vi "ErrorDialog.vi"(8 "error in":errorcluster) -> (0 "error out":errorcluster)   [LabVIEW 2010]
panel:
  out "Message":string
  in  "OK":bool
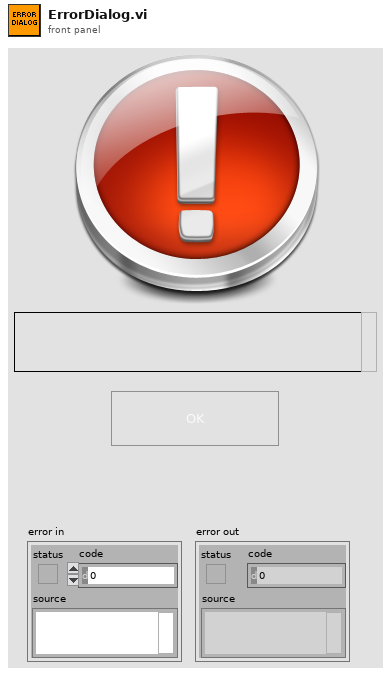
[diagram p1: front panel]
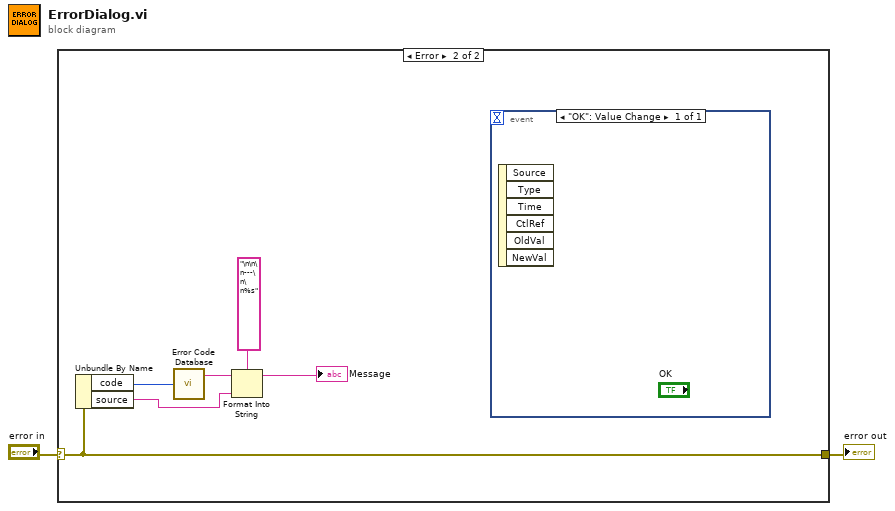
[diagram p0: block diagram]
diagram:
  n1 = case shown="Error" "error in" {
    selector: "error in" -> [w3 w9]
    tunnel: [w3 w9] -> w1
    frame No Error {
    }
    frame Error {
      n2 = Unbundle By Name(w9) -> ("code"=w8:i32, "source"=w4:string)
      n3 = call <vilib>:"Error Code Database.vi"("Error Code"=w8) -> ("Error Text"=w7:string)
      n4 = Format Into String(format string="\n\n\n---\n\n%s", initial string=w7, w4) -> (resulting string=→"Message":string)  [unwired: 1 in, 1 out]
      n5 = event shown="[0] \"OK\": Value Change" {
        selector: _ -> [_]
        dyn-events: _ -> [_]
        timeout: _ -> [_]
        event "OK": Value Change {
          n6 = event-data() -> ()  [unwired: 7 out]
        }
      }
    }
  }
  "error out" <- w1
